vi "_MenuVIs.vi"() -> (3 "VIs":refnum<vi>[](array[refnum]))   [LabVIEW 2017, in "tagdb-RefMgr Operations.lvlib"]
uses:
  tagdb-RefMgr Operations.lvlib
  Menu_Check.vi
  Menu_Disable.vi
  Menu_Enable.vi
  Menu_ItemName.vi
  Menu_ToggleCheck.vi
  Menu_ToggleEnable.vi
  Menu_unCheck.vi
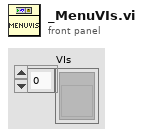
[diagram p1: front panel]
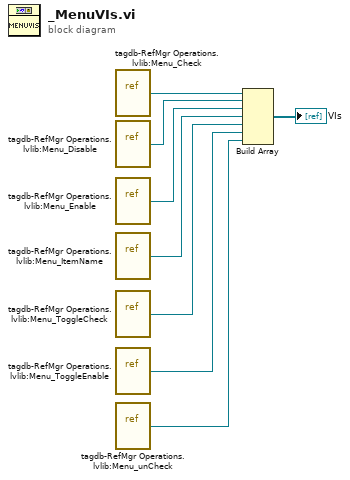
[diagram p0: block diagram]
diagram:
  n1 = vi-ref "tagdb-RefMgr Operations.lvlib:Menu_Check.vi"() -> (w3:refnum<vi>)
  n2 = vi-ref "tagdb-RefMgr Operations.lvlib:Menu_Disable.vi"() -> (w4:refnum<vi>)
  n3 = vi-ref "tagdb-RefMgr Operations.lvlib:Menu_Enable.vi"() -> (w5:refnum<vi>)
  n4 = vi-ref "tagdb-RefMgr Operations.lvlib:Menu_ItemName.vi"() -> (w6:refnum<vi>)
  n5 = vi-ref "tagdb-RefMgr Operations.lvlib:Menu_ToggleCheck.vi"() -> (w7:refnum<vi>)
  n6 = vi-ref "tagdb-RefMgr Operations.lvlib:Menu_ToggleEnable.vi"() -> (w8:refnum<vi>)
  n7 = vi-ref "tagdb-RefMgr Operations.lvlib:Menu_unCheck.vi"() -> (w2:refnum<vi>)
  n8 = Build Array(w3, w4, w5, w6, w7, w8, w2) -> (→"VIs":refnum<vi>[])
